vi "UsesTypeDef.vi"() -> ()   [LabVIEW 2020]
uses:
  Typedef.ctl
panel:
  in  "Cluster":T1
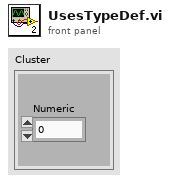
[diagram p1: front panel]
types:
  T1 = typedef "Typedef.ctl" = cluster{"Numeric":dbl}
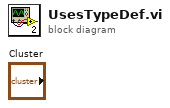
[diagram p0: block diagram]
diagram:
